vi "AddfourierComposant.vi"(8 "disabled index (col)":i32, 9 "index (row)":i32, 10 "?":dbl format="%#_13g", 11 "FFT matrix":dbl[][](array[numeric])) -> (3 "output array":dbl[][](array[numeric]))   [LabVIEW 2015]
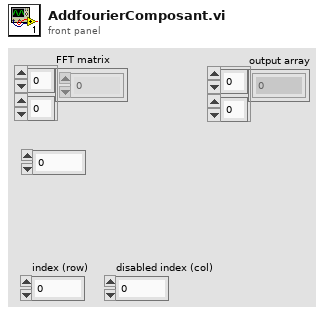
[diagram p1: front panel]
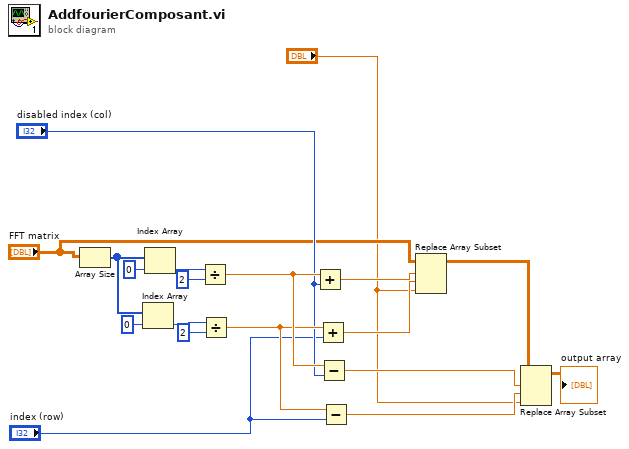
[diagram p0: block diagram]
diagram:
  n1 = Array Size(array="FFT matrix") -> (size(s)=w19:i32[])
  n2 = Index Array(array=w19, index=0) -> (element=w14:i32)
  n3 = Index Array(array=w19, index=0) -> (element=w16:i32)
  n4 = Divide(x=w16, y=2) -> (x/y=w10:dbl)
  n5 = Divide(x=w14, y=2) -> (x/y=w9:dbl)
  n6 = Add(x=w10, y="disabled index (col)") -> (x+y=w12:dbl)
  n7 = Add(x=w9, y="index (row)") -> (x+y=w11:dbl)
  n8 = Subtract(x=w10, y="disabled index (col)") -> (x-y=w5:dbl)
  n9 = Subtract(x=w9, y="index (row)") -> (x-y=w6:dbl)
  n10 = Replace Array Subset(array="FFT matrix", new element="?", index (row)=w12, index (col)=w11) -> (w3:dbl[][])
  n11 = Replace Array Subset(array=w3, new element="?", index (row)=w5, index (col)=w6) -> (→"output array":dbl[][])
